vi "Set Starter Motor Duty Cycle.vi"(8 "Error In":errorcluster, 10 "Duty Cycle":i32, 11 "ECU COM Port":refnum<visa-resource-name>) -> (0 "Error Out":errorcluster, 3 "ECU COM Port Out":refnum<visa-resource-name>)   [LabVIEW 2017]
doc: "<b>Description</b>\nThis VI sets the duty cycle of the starter motor.\n\n<b>Inputs</b>\nECU COM Port: The com port of the ECU.\nDuty Cycle: The desired duty cycle of the starter motor. This is a number between 0-20, where each integer increment represents a 5% step in duty cycle.\n\n<b>Outputs</b>\nECU COM Port Out: The com port of the ECU."
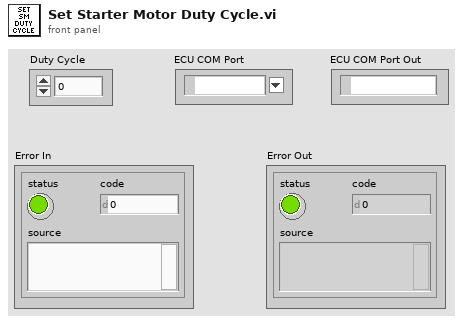
[diagram p1: front panel]
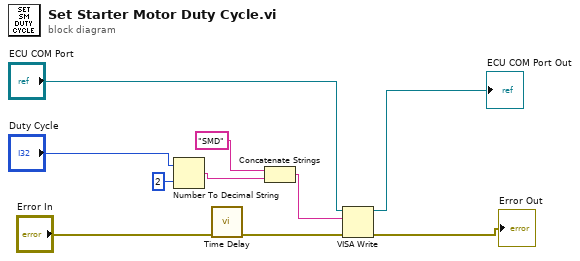
[diagram p0: block diagram]
diagram:
  n1 = Number To Decimal String(number="Duty Cycle", width (-)=i16 2) -> (decimal integer string=w9:string)
  n2 = call "Time Delay"("error in (no error)"="Error In") -> ("error out"=w2:errorcluster)  [unwired: 10 in]
  n3 = Concatenate Strings("SMD" ("write buffer"), w9) -> (w10:string)
  n4 = VISA Write(VISA resource name="ECU COM Port", write buffer=w10, error in (no error)=w2) -> (VISA resource name out=→"ECU COM Port Out":refnum<visa-resource-name>, error out=→"Error Out":errorcluster)  [unwired: 1 out]
